vi "加标回收参数设置.vi"() -> ()   [LabVIEW 2016, in "质控单元V4.lvlib"]
panel:
  in  "显示详细日志":bool
  in  "布尔":bool
  in  "Tab Control 2":enum32{"氨氮", "总磷", "总氮", "高锰酸盐指数", "化学需氧量"}(tab)
  in  "启用":bool
  out "氨氮加标回收率":sgl caption="加标回收率" format="%#.2f"
  out "氨氮加标体积":sgl caption="加标体积" format="%#.4f"
  in  "氨氮母液浓度":sgl caption="母液浓度"
  in  "氨氮定容体积":sgl caption="定容体积"
  out "氨氮加标后水样浓度":sgl caption="加标后水样浓度" format="%#.4f"
  out "氨氮加标前水样浓度":sgl caption="加标前水样浓度" format="%#.4f"
  in  "氨氮量程":sgl caption="量程"
  in  "氨氮检出限":sgl caption="检出限"
  in  "启用 2":bool
  out "TP加标回收率":sgl caption="加标回收率" format="%#.2f"
  out "TP加标体积":sgl caption="加标体积" format="%#.4f"
  in  "TP母液浓度":sgl caption="母液浓度"
  in  "TP定容体积":sgl caption="定容体积"
  out "TP加标后水样浓度":sgl caption="加标后水样浓度" format="%#.4f"
  out "TP加标前水样浓度":sgl caption="加标前水样浓度" format="%#.4g"
  in  "TP量程":sgl caption="量程"
  in  "TP检出限":sgl caption="检出限"
  in  "启用 3":bool
  out "TN加标回收率":sgl caption="加标回收率" format="%#.2f"
  out "TN加标体积":sgl caption="加标体积" format="%#.4f"
  in  "TN母液浓度":sgl caption="母液浓度"
  in  "TN定容体积":sgl caption="定容体积"
  out "TN加标后水样浓度":sgl caption="加标后水样浓度" format="%#.4f"
  out "TN加标前水样浓度":sgl caption="加标前水样浓度" format="%#.4f"
  in  "TN量程":sgl caption="量程"
  in  "TN检出限":sgl caption="检出限"
  in  "启用 4":bool
  out "CODMn加标回收率":sgl caption="加标回收率" format="%#.2f"
  out "CODMn加标体积":sgl caption="加标体积" format="%#.4f"
  in  "CODMn母液浓度":sgl caption="母液浓度"
  in  "CODMn定容体积":sgl caption="定容体积"
  out "CODMn加标后水样浓度":sgl caption="加标后水样浓度" format="%#.4f"
  out "CODMn加标前水样浓度":sgl caption="加标前水样浓度" format="%#.4f"
  in  "CODMn量程":sgl caption="量程"
  in  "CODMn检出限":sgl caption="检出限"
  in  "启用 5":bool
  out "CODCr加标回收率":sgl caption="加标回收率" format="%#.2f"
  out "CODCr加标体积":sgl caption="加标体积" format="%#.4f"
  in  "CODCr母液浓度":sgl caption="母液浓度"
  in  "CODCr定容体积":sgl caption="定容体积"
  out "CODCr加标后水样浓度":sgl caption="加标后水样浓度" format="%#.4f"
  out "CODCr加标前水样浓度":sgl caption="加标前水样浓度" format="%#.4f"
  in  "CODCr量程":sgl caption="量程"
  in  "CODCr检出限":sgl caption="检出限"
  # "加标回收参数设置"
  # "加标回收参数"
  # "加标回收参数"
  # "加标回收参数"
  # "加标回收参数"
  # "加标回收参数"
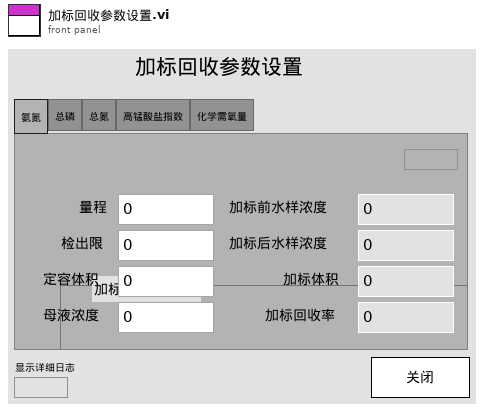
[diagram p1: front panel]
types:
  T1 = cluster{"氨氮":bool, "总磷":bool, "总氮":bool, "CODMn":bool, "CODCr":bool}
  T2 = cluster{"量程":dbl, "检出限":dbl, "加标前水样浓度":dbl, "加标后水样浓度":dbl, "加标水杯定容体积":dbl, "加标母液浓度":dbl, "加标体积":dbl, "加标回收率":dbl}
  T3 = cluster{"氨氮":bool, "总磷":bool, "总氮":bool, "CODMn":bool, "CODCr":bool, "氨氮总磷":bool, "总磷总氮":bool}
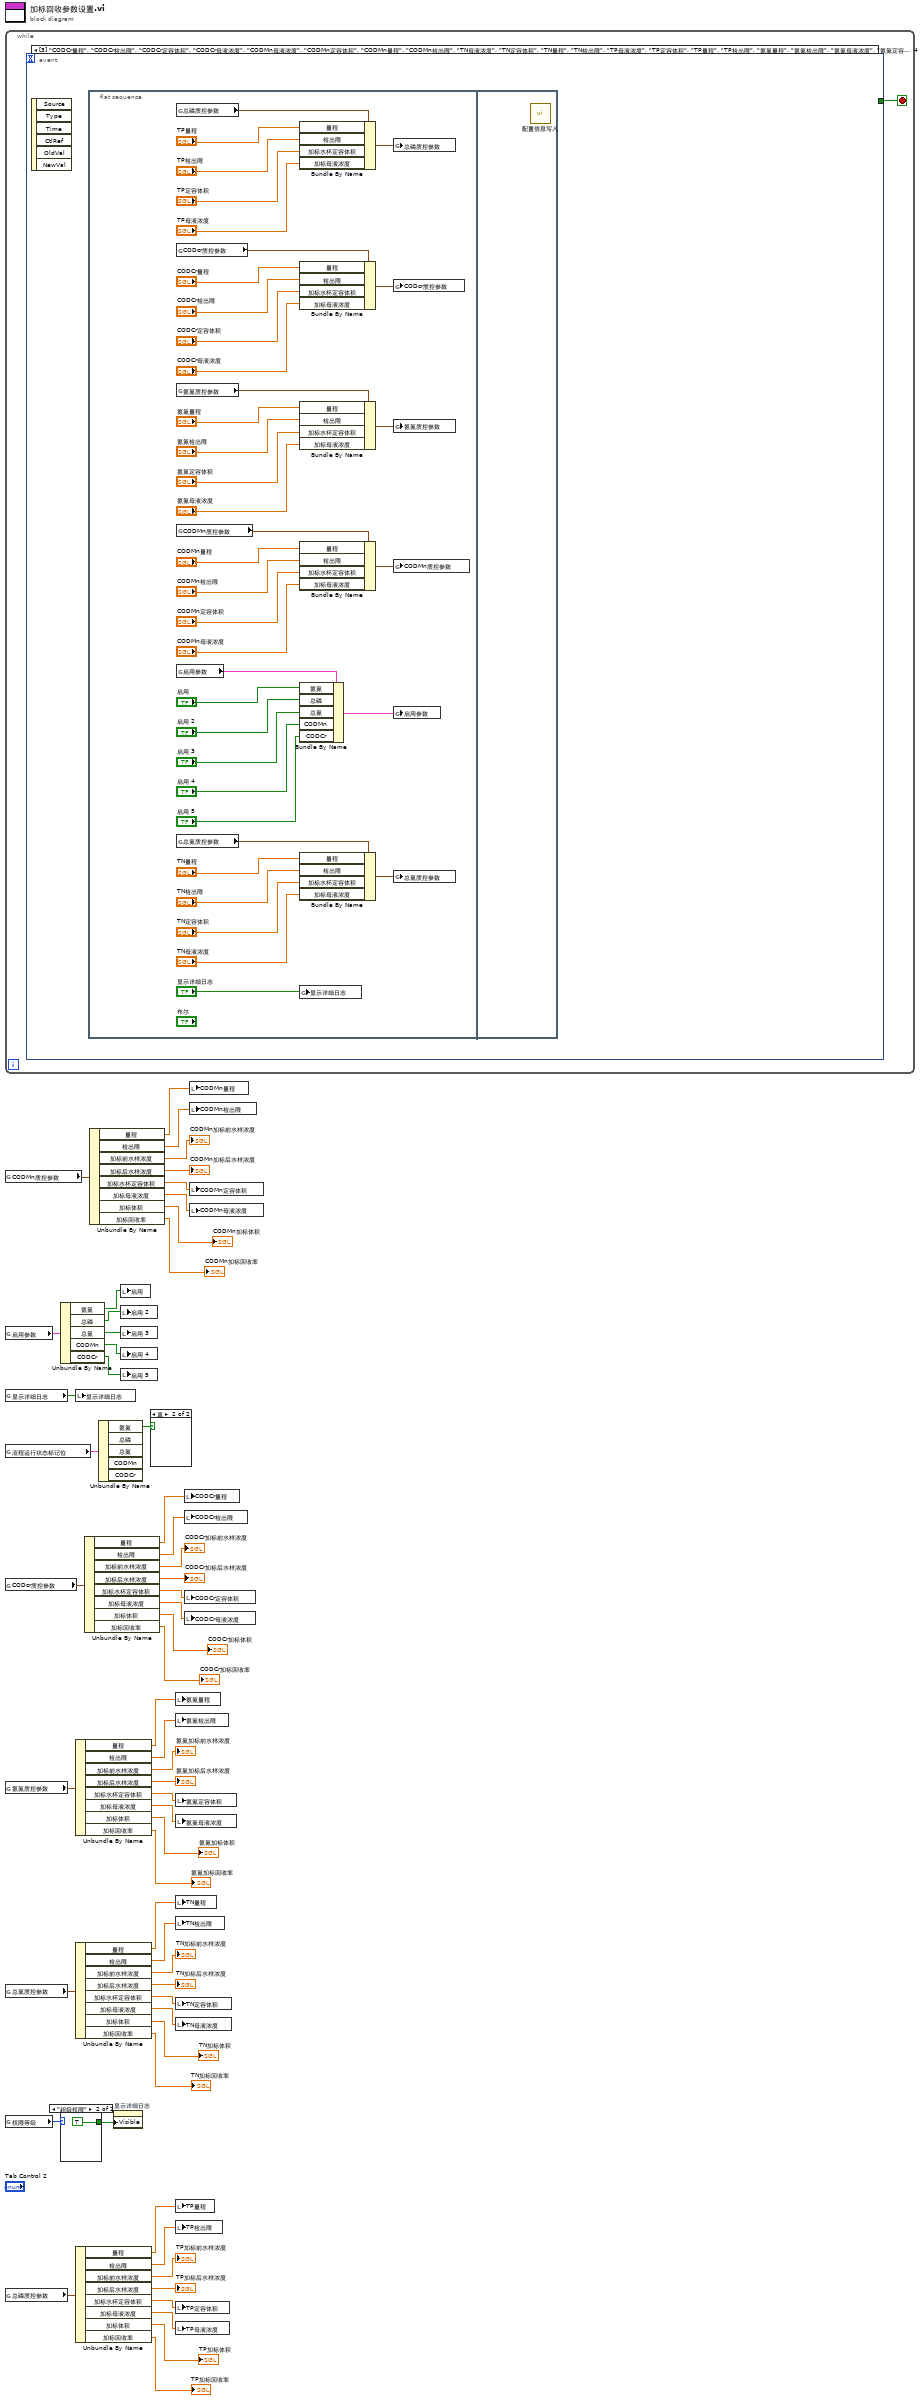
[diagram p0: block diagram]
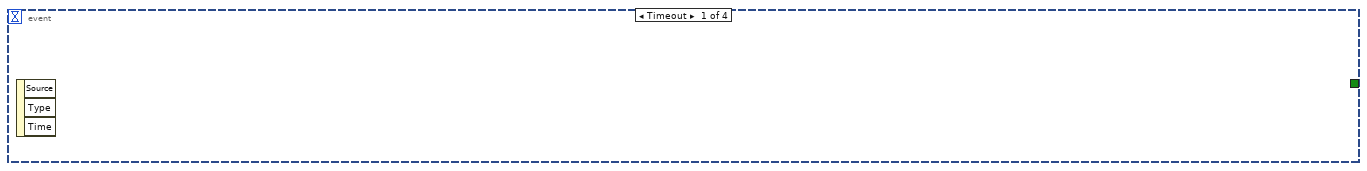
[diagram p4: hidden frame]
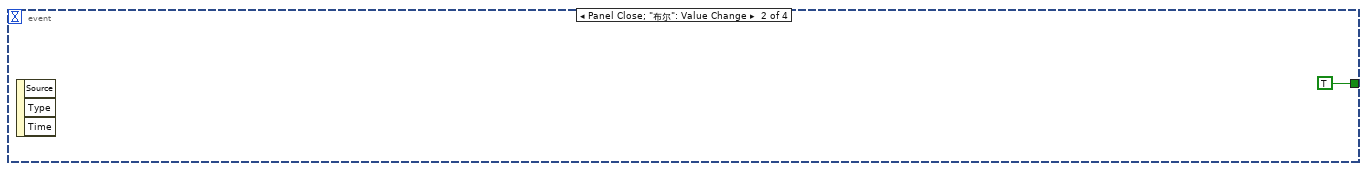
[diagram p5: hidden frame]
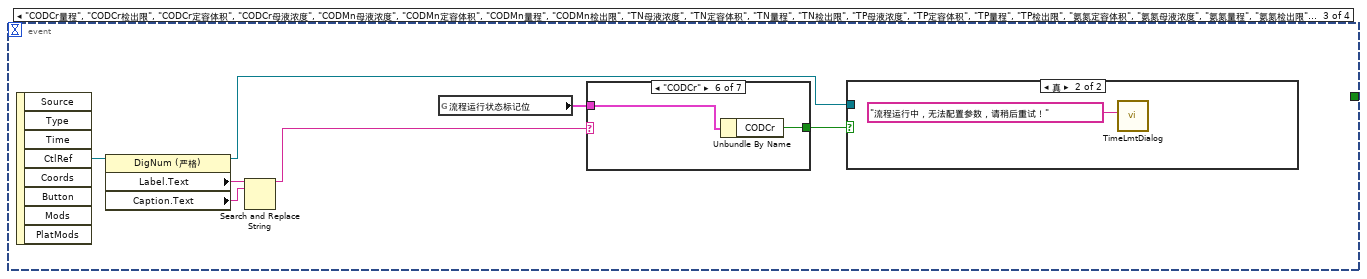
[diagram p6: hidden frame]
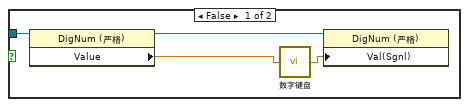
[diagram p7: hidden frame]
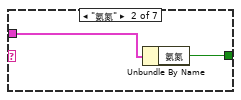
[diagram p9: hidden frame]
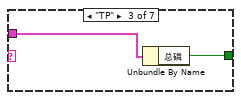
[diagram p10: hidden frame]
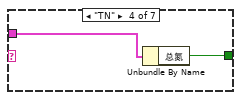
[diagram p11: hidden frame]
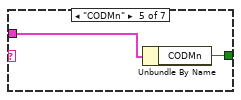
[diagram p12: hidden frame]
diagram:
  n1 = while {
    stop <- w57 stop-if-true
    n2 = event shown="[3] \"CODCr量程\", \"CODCr检出限\", \"CODCr定容体积\", \"CODCr母液浓度\", \"CODMn母液浓度\", \"CODMn定容体积\", \"CODMn量程\", \"CODMn检出限\", \"TN母液浓度\", \"TN定容体积\", \"TN量程\", \"TN检出限\", \"TP母液浓度\", \"TP定容体积\", \"TP量程\", \"TP检出限\", \"氨氮量程\", \"氨氮检出限\", \"氨氮母液浓度\", \"氨氮定容体积\", \"启用\", \"启用 2\", \"启用 3\", \"启用 4\", \"启用 5\": 值改变" {
      selector: _ -> [_ _ _ _]
      dyn-events: _ -> [_ _ _ _]
      timeout: _ -> [_ _ _ _]
      tunnel: [_ TRUE _ _] -> w57
      event Timeout {
        n3 = event-data() -> ()  [unwired: 1 in, 3 out]
      }
      event Panel Close; "布尔": Value Change {
        n4 = event-data() -> ()  [unwired: 1 in, 3 out]
      }
      event "CODCr量程", "CODCr检出限", "CODCr定容体积", "CODCr母液浓度", "CODMn母液浓度", "CODMn定容体积", "CODMn量程", "CODMn检出限", "TN母液浓度", "TN定容体积", "TN量程", "TN检出限", "TP母液浓度", "TP定容体积", "TP量程", "TP检出限", "氨氮定容体积", "氨氮母液浓度", "氨氮量程", "氨氮检出限": Mouse Down {
        n5 = event-data() -> ("CtlRef"=w65:refnum<vi>)  [unwired: 1 in, 7 out]
        n6 = property class="DigNum (严格)"(reference=w65) -> (reference out=w64:refnum<vi>, "Label.Text"=w63:string, "Caption.Text"=w62:string)  [unwired: 1 in, 1 out]
        n7 = Search and Replace String(input string=w63, search string=w62) -> (result string=w61:string)  [unwired: 6 in, 3 out]
        n8 = global read "ZK非断电保存全局变量.vi" "流程运行状态标记位"() -> (w60:T1)
        n9 = case shown="\"CODCr\"" w61 {
          tunnel: w60 -> [_ w72 w74 w76 w78 w80 _]
          tunnel: [_ w71 w73 w75 w77 w79 _] -> w59
          frame Default {
          }
          frame "氨氮" {
            n10 = Unbundle By Name(w72) -> ("氨氮"=w71:bool)
          }
          frame "TP" {
            n11 = Unbundle By Name(w74) -> ("总磷"=w73:bool)
          }
          frame "TN" {
            n12 = Unbundle By Name(w76) -> ("总氮"=w75:bool)
          }
          frame "CODMn" {
            n13 = Unbundle By Name(w78) -> ("CODMn"=w77:bool)
          }
          frame "CODCr" {
            n14 = Unbundle By Name(w80) -> ("CODCr"=w79:bool)
          }
          frame "真" {
          }
        }
        n15 = case shown="真" w59 {
          tunnel: w64 -> [w66 _]
          frame False {
            n16 = property class="DigNum (严格)"(reference=w66) -> (reference out=w68:refnum<vi>, "Value"=w69:sgl)  [unwired: 1 in, 1 out]
            n17 = call "数字键盘.vi"("OldNumber"=w69) -> ("NewNumber"=w67:sgl)
            n18 = property class="DigNum (严格)"(reference=w68, "Val(Sgnl)"=w67) -> ()  [unwired: 1 in, 2 out]
          }
          frame True {
            n19 = call "TimeLmtDialog.vi"("Infoin"="流程运行中，无法配置参数，请稍后重试！") -> ()  [unwired: 11 in]
          }
        }
      }
      event "CODCr量程", "CODCr检出限", "CODCr定容体积", "CODCr母液浓度", "CODMn母液浓度", "CODMn定容体积", "CODMn量程", "CODMn检出限", "TN母液浓度", "TN定容体积", "TN量程", "TN检出限", "TP母液浓度", "TP定容体积", "TP量程", "TP检出限", "氨氮量程", "氨氮检出限", "氨氮母液浓度", "氨氮定容体积", "启用", "启用 2", "启用 3", "启用 4", "启用 5": Value Change {
        n20 = event-data() -> ()  [unwired: 1 in, 6 out]
        n21 = flat-sequence {
          frame #0 {
            n22 = global read "ZK断电保存全局变量.vi" "总磷质控参数"() -> (w94:T2)
            n23 = global read "ZK断电保存全局变量.vi" "CODcr质控参数"() -> (w111:T2)
            n24 = global read "ZK断电保存全局变量.vi" "氨氮质控参数"() -> (w106:T2)
            n25 = global read "ZK断电保存全局变量.vi" "CODMn质控参数"() -> (w118:T2)
            n26 = global read "ZK断电保存全局变量.vi" "启用参数"() -> (w88:T3)
            n27 = global read "ZK断电保存全局变量.vi" "总氮质控参数"() -> (w99:T2)
            n28 = Bundle By Name(cluster=w94, "量程"="TP量程", "检出限"="TP检出限", "加标水杯定容体积"="TP定容体积", "加标母液浓度"="TP母液浓度") -> (w93:T2)
            n29 = Bundle By Name(cluster=w111, "量程"="CODCr量程", "检出限"="CODCr检出限", "加标水杯定容体积"="CODCr定容体积", "加标母液浓度"="CODCr母液浓度") -> (w112:T2)
            n30 = Bundle By Name(cluster=w106, "量程"="氨氮量程", "检出限"="氨氮检出限", "加标水杯定容体积"="氨氮定容体积", "加标母液浓度"="氨氮母液浓度") -> (w105:T2)
            n31 = Bundle By Name(cluster=w118, "量程"="CODMn量程", "检出限"="CODMn检出限", "加标水杯定容体积"="CODMn定容体积", "加标母液浓度"="CODMn母液浓度") -> (w117:T2)
            n32 = Bundle By Name(cluster=w88, "氨氮"="启用", "总磷"="启用 2", "总氮"="启用 3", "CODMn"="启用 4", "CODCr"="启用 5") -> (w87:T3)
            n33 = Bundle By Name(cluster=w99, "量程"="TN量程", "检出限"="TN检出限", "加标水杯定容体积"="TN定容体积", "加标母液浓度"="TN母液浓度") -> (w100:T2)
            n34 = global write "ZK断电保存全局变量.vi" "显示详细日志"("显示详细日志") -> ()
            n35 = global write "ZK断电保存全局变量.vi" "总磷质控参数"(w93) -> ()
            n36 = global write "ZK断电保存全局变量.vi" "CODcr质控参数"(w112) -> ()
            n37 = global write "ZK断电保存全局变量.vi" "氨氮质控参数"(w105) -> ()
            n38 = global write "ZK断电保存全局变量.vi" "CODMn质控参数"(w117) -> ()
            n39 = global write "ZK断电保存全局变量.vi" "启用参数"(w87) -> ()
            n40 = global write "ZK断电保存全局变量.vi" "总氮质控参数"(w100) -> ()
          }
          frame #1 {
            n41 = call "配置信息写入.vi"() -> ()  [unwired: 11 in, 1 out]
          }
        }
      }
    }
  }
  n42 = global read "ZK断电保存全局变量.vi" "CODMn质控参数"() -> (w56:T2)
  n43 = global read "ZK断电保存全局变量.vi" "启用参数"() -> (w9:T3)
  n44 = global read "ZK断电保存全局变量.vi" "显示详细日志"() -> (w3:bool)
  n45 = global read "ZK非断电保存全局变量.vi" "流程运行状态标记位"() -> (w11:T1)
  n46 = global read "ZK断电保存全局变量.vi" "CODcr质控参数"() -> (w47:T2)
  n47 = global read "ZK断电保存全局变量.vi" "氨氮质控参数"() -> (w38:T2)
  n48 = global read "ZK断电保存全局变量.vi" "总氮质控参数"() -> (w29:T2)
  n49 = global read "ZK非断电保存全局变量.vi" "权限等级"() -> (w2:enum16{"一级权限", "二级权限", "三级权限", "超级权限"})
  n50 = global read "ZK断电保存全局变量.vi" "总磷质控参数"() -> (w27:T2)
  n51 = Unbundle By Name(w9) -> ("氨氮"=w8:bool, "总磷"=w7:bool, "总氮"=w6:bool, "CODMn"=w5:bool, "CODCr"=w4:bool)
  n52 = case shown="\"超级权限\"" w2 {
    tunnel: [_ TRUE] -> w1
    frame "一级权限", Default {
    }
    frame "超级权限" {
    }
  }
  n53 = local write "显示详细日志"(w3) -> ()
  n54 = Unbundle By Name(w38) -> ("量程"=w33:dbl, "检出限"=w32:dbl, "加标前水样浓度"=→"氨氮加标前水样浓度":dbl, "加标后水样浓度"=→"氨氮加标后水样浓度":dbl, "加标水杯定容体积"=w31:dbl, "加标母液浓度"=w30:dbl, "加标体积"=→"氨氮加标体积":dbl, "加标回收率"=→"氨氮加标回收率":dbl)
  n55 = Unbundle By Name(w29) -> ("量程"=w15:dbl, "检出限"=w14:dbl, "加标前水样浓度"=→"TN加标前水样浓度":dbl, "加标后水样浓度"=→"TN加标后水样浓度":dbl, "加标水杯定容体积"=w13:dbl, "加标母液浓度"=w12:dbl, "加标体积"=→"TN加标体积":dbl, "加标回收率"=→"TN加标回收率":dbl)
  n56 = Unbundle By Name(w27) -> ("量程"=w19:dbl, "检出限"=w18:dbl, "加标前水样浓度"=→"TP加标前水样浓度":dbl, "加标后水样浓度"=→"TP加标后水样浓度":dbl, "加标水杯定容体积"=w17:dbl, "加标母液浓度"=w16:dbl, "加标体积"=→"TP加标体积":dbl, "加标回收率"=→"TP加标回收率":dbl)
  n57 = Unbundle By Name(w47) -> ("量程"=w42:dbl, "检出限"=w41:dbl, "加标前水样浓度"=→"CODCr加标前水样浓度":dbl, "加标后水样浓度"=→"CODCr加标后水样浓度":dbl, "加标水杯定容体积"=w40:dbl, "加标母液浓度"=w39:dbl, "加标体积"=→"CODCr加标体积":dbl, "加标回收率"=→"CODCr加标回收率":dbl)
  n58 = Unbundle By Name(w56) -> ("量程"=w51:dbl, "检出限"=w50:dbl, "加标前水样浓度"=→"CODMn加标前水样浓度":dbl, "加标后水样浓度"=→"CODMn加标后水样浓度":dbl, "加标水杯定容体积"=w49:dbl, "加标母液浓度"=w48:dbl, "加标体积"=→"CODMn加标体积":dbl, "加标回收率"=→"CODMn加标回收率":dbl)
  n59 = Unbundle By Name(w11) -> ("氨氮"=w10:bool)  [unwired: 4 out]
  n60 = property on="显示详细日志" class="Bool (严格)"("Visible"=w1) -> ()  [unwired: 2 in, 2 out]
  n61 = local write "启用"(w8) -> ()
  n62 = local write "启用 2"(w7) -> ()
  n63 = local write "启用 3"(w6) -> ()
  n64 = local write "启用 4"(w5) -> ()
  n65 = local write "启用 5"(w4) -> ()
  n66 = case shown="真" w10 {
    frame False {
    }
    frame True {
    }
  }
  n67 = local write "氨氮量程"(w33) -> ()
  n68 = local write "氨氮检出限"(w32) -> ()
  n69 = local write "氨氮定容体积"(w31) -> ()
  n70 = local write "氨氮母液浓度"(w30) -> ()
  n71 = local write "TN量程"(w15) -> ()
  n72 = local write "TN检出限"(w14) -> ()
  n73 = local write "TN定容体积"(w13) -> ()
  n74 = local write "TN母液浓度"(w12) -> ()
  n75 = local write "TP量程"(w19) -> ()
  n76 = local write "TP检出限"(w18) -> ()
  n77 = local write "TP定容体积"(w17) -> ()
  n78 = local write "TP母液浓度"(w16) -> ()
  n79 = local write "CODCr量程"(w42) -> ()
  n80 = local write "CODCr检出限"(w41) -> ()
  n81 = local write "CODCr定容体积"(w40) -> ()
  n82 = local write "CODCr母液浓度"(w39) -> ()
  n83 = local write "CODMn量程"(w51) -> ()
  n84 = local write "CODMn检出限"(w50) -> ()
  n85 = local write "CODMn定容体积"(w49) -> ()
  n86 = local write "CODMn母液浓度"(w48) -> ()
